vi "Get ni_bus_monitor_api_InitializeSettingsRequest.vi"(8 "error in (no error)":errorcluster, 11 "gRPCid":T1) -> (0 "error out":errorcluster, 2 "package_templatemessage":T2, 3 "gRPCid out":T1)   [LabVIEW 2025, in "bus_monitor_server.lvlib"]
uses:
  bus_monitor_server.lvlib
  ni_bus_monitor_api_InitializeSettingsRequest.ctl
  ni_bus_monitor_api_ConnectSettings.ctl
  ni_bus_monitor_api_CanMode.ctl
  ni_bus_monitor_api_Termination.ctl
  ni_bus_monitor_api_FdIsoMode.ctl
  <vilib>/gRPC/LabVIEW gRPC Library/Shared/grpcId.ctl
  ni_bus_monitor_api_InitializeSettingsRequest_Flat.ctl
  ni_bus_monitor_api_ConnectSettings_Flat.ctl
  2ed25e12-861d-4677-8ead-ace2906b2041.vi
  <vilib>/gRPC/LabVIEW gRPC Library/Shared/TranslateGrpcError.vi
  FlatToRichni_bus_monitor_api_ConnectSettings.vi
  <vilib>/gRPC/LabVIEW gRPC Library/Server API/Server/Get Server DLL Path.vi
  <vilib>/Utility/error.llb/Error Cluster From Error Code.vi
  <vilib>/gRPC/LabVIEW gRPC Library/grpc-lvsupport-release.lvlib
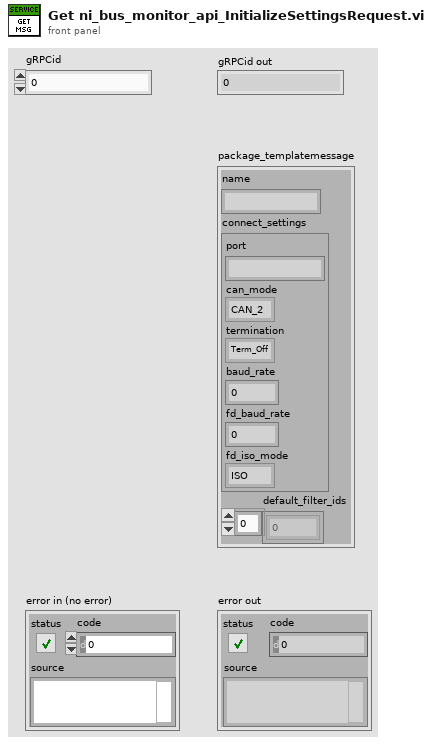
[diagram p1: front panel]
types:
  T1 = typedef "grpc-lvsupport-release.lvlib/grpcId.ctl" = u64
  T2 = typedef "bus_monitor_server.lvlib/ni_bus_monitor_api_InitializeSettingsRequest.ctl" = cluster{"name":string, "connect_settings":T3, "default_filter_ids":u32[]}
  T3 = typedef "bus_monitor_server.lvlib/ni_bus_monitor_api_ConnectSettings.ctl" = cluster{"port":string, "can_mode":T4, "termination":T5, "baud_rate":u64, "fd_baud_rate":u64, "fd_iso_mode":T6}
  T4 = typedef "bus_monitor_server.lvlib/ni_bus_monitor_api_CanMode.ctl" = enum32{"CAN_2", "CAN_FD", "CAN_FD_BRS"}
  T5 = typedef "bus_monitor_server.lvlib/ni_bus_monitor_api_Termination.ctl" = enum32{"Term_Off", "Term_On"}
  T6 = typedef "bus_monitor_server.lvlib/ni_bus_monitor_api_FdIsoMode.ctl" = enum32{"ISO", "Non_ISO", "ISO_Legacy"}
  T7 = typedef "bus_monitor_server.lvlib/ni_bus_monitor_api_InitializeSettingsRequest_Flat.ctl" = cluster{"name":string, "connect_settings":T8, "default_filter_ids":u32[]}
  T8 = typedef "bus_monitor_server.lvlib/ni_bus_monitor_api_ConnectSettings_Flat.ctl" = cluster{"port":string, "can_mode":T4, "termination":T5, "baud_rate":u64, "fd_baud_rate":u64, "fd_iso_mode":T6}
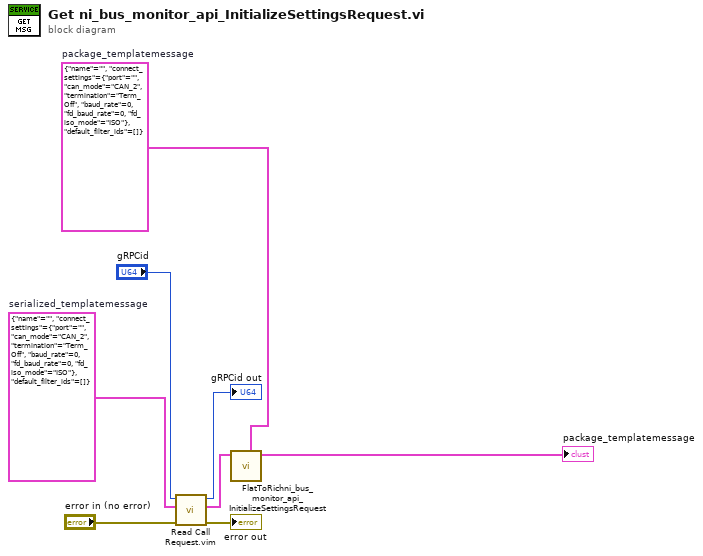
[diagram p0: block diagram]
diagram:
  w6 = T7 {"name"="", "connect_settings"={"port"="", "can_mode"=enum."CAN_2", "termination"=enum."Term_Off", "baud_rate"=0, "fd_baud_rate"=0, "fd_iso_mode"=enum."ISO"}, "default_filter_ids"=[]}  # serialized_templatemessage
  w5 = T2 {"name"="", "connect_settings"={"port"="", "can_mode"=enum."CAN_2", "termination"=enum."Term_Off", "baud_rate"=0, "fd_baud_rate"=0, "fd_iso_mode"=enum."ISO"}, "default_filter_ids"=[]}  # package_templatemessage
  n1 = call "Read Call Request.vim"("error in"="error in (no error)", "Request Type"=w6, "gRPCid in"="gRPCid") -> ("error out"=→"error out":errorcluster, "Request Data"=w4:T7, "gRPCid out"=→"gRPCid out":T1)  [unwired: 6 in]
  n2 = call "FlatToRichni_bus_monitor_api_InitializeSettingsRequest.vi"("OutputClusterType"=w5, "InputCluster"=w4) -> ("OutputCluster"=→"package_templatemessage":T2)  [unwired: 9 in]
